vi "2L16_2D_carte_m_de_lim_et_moyech_.vi"(9 "Moyennes éch.":dbl[](array[numeric]), 10 "Limites contrôle":dbl[](array[numeric]), 11 "Limite alerte":dbl[](array[numeric])) -> (3 "Moyennes + limites":dbl[][](array[numeric]))   [LabVIEW 2010, in "lv_02.lvlib"]
uses:
  lv_02.lvlib
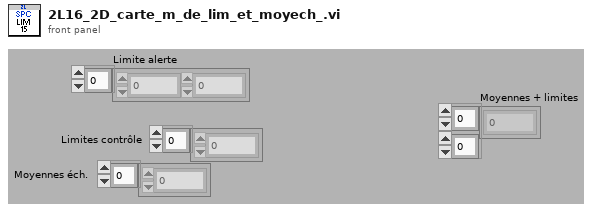
[diagram p1: front panel]
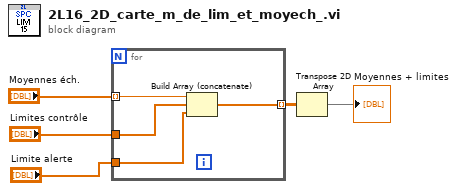
[diagram p0: block diagram]
diagram:
  n1 = for {
    tunnel: "Moyennes éch." -> [w9] mode=indexing
    tunnel: "Limites contrôle" -> [w8]
    tunnel: "Limite alerte" -> [w7]
    tunnel: [w6] -> w2 mode=indexing
    n2 = Build Array (concatenate)(w9, w8, w7) -> (w6:dbl[])
  }
  n3 = Transpose 2D Array(2D array=w2) -> (transposed array=→"Moyennes + limites":dbl[][])
